vi "X_C_4352_15.vi"(0 "ek":dbl format="%#_13g", 2 "length":i32=15, 3 "q":dbl[](array[numeric])=[1.0, 1.0, 1.0, 1.0, 1.0, 1.0, 1.0, 1.0, 1.0, 1.0, 1.0, 1.0, 1.0, 1.0, 1.0] format="%#_13g") -> (5 "uk":dbl format="%#_13g")   [LabVIEW 2015]
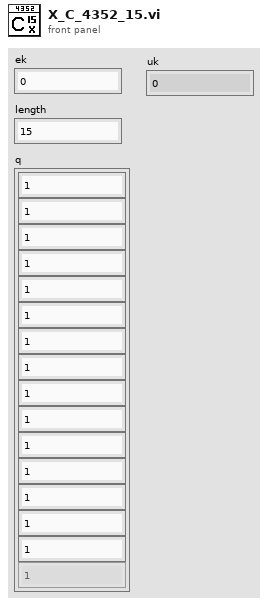
[diagram p1: front panel]
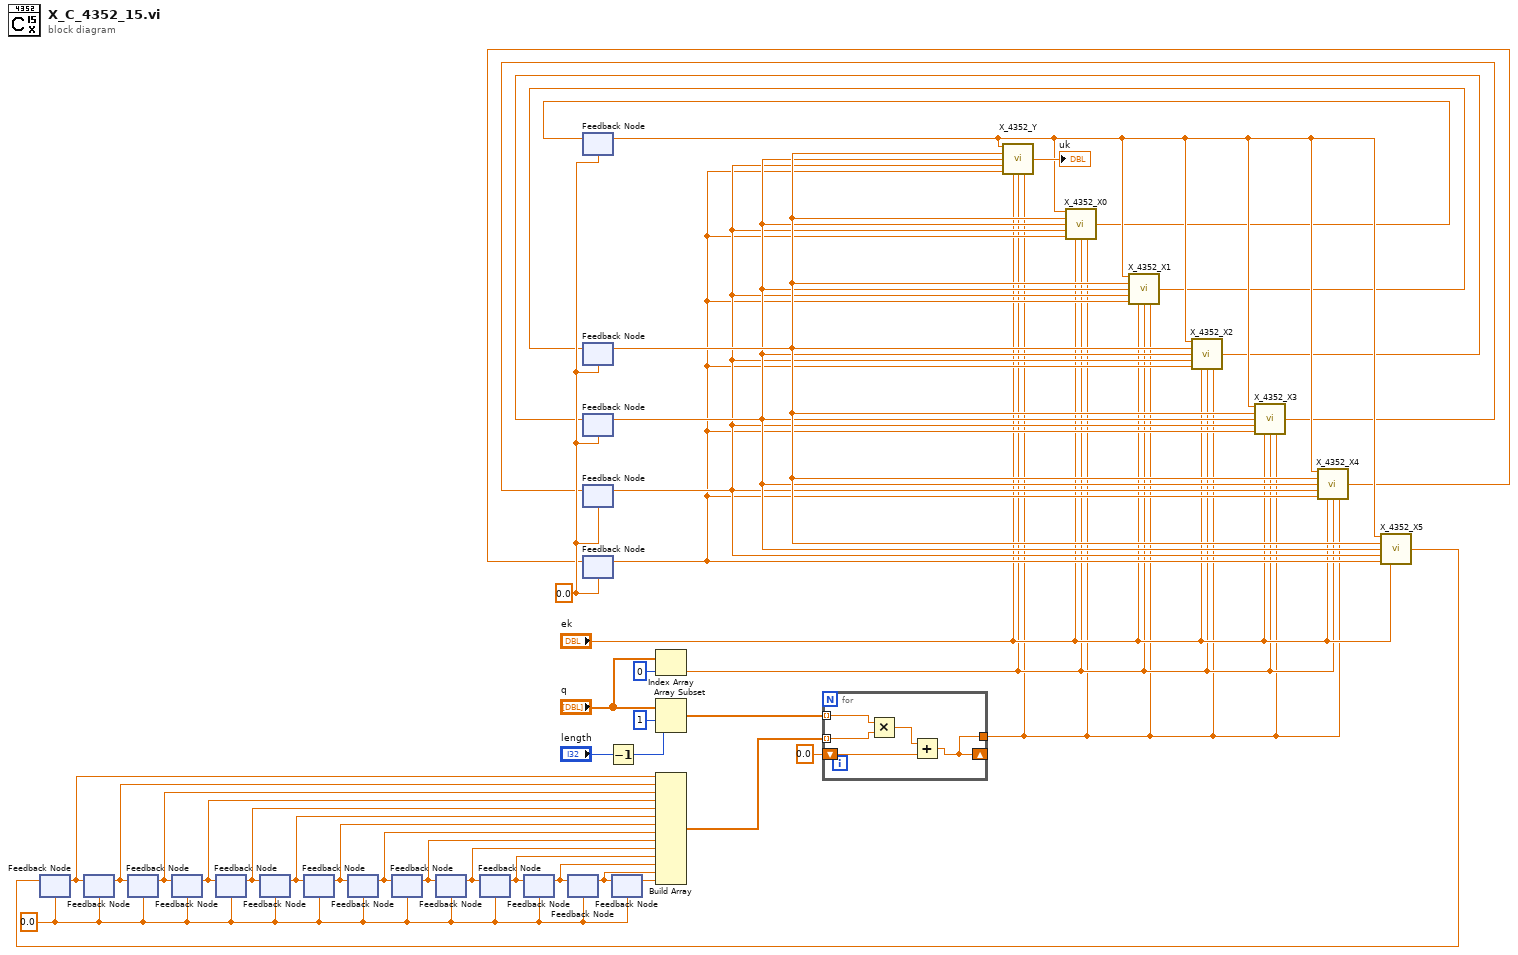
[diagram p0: block diagram]
diagram:
  w17 = 0.0
  w32 = 0.0
  n1 = feedback #1(w17) -> (w18:dbl)
  n2 = feedback #2(w17) -> (w19:dbl)
  n3 = feedback-in #2(w18) -> ()
  n4 = feedback #3(w17) -> (w20:dbl)
  n5 = feedback-in #3(w19) -> ()
  n6 = feedback #4(w17) -> (w21:dbl)
  n7 = feedback-in #4(w20) -> ()
  n8 = feedback #5(w17) -> (w22:dbl)
  n9 = feedback-in #5(w21) -> ()
  n10 = feedback #6(w17) -> (w23:dbl)
  n11 = feedback-in #6(w22) -> ()
  n12 = feedback #7(w17) -> (w24:dbl)
  n13 = feedback-in #7(w23) -> ()
  n14 = feedback #8(w17) -> (w25:dbl)
  n15 = feedback-in #8(w24) -> ()
  n16 = feedback #9(w17) -> (w26:dbl)
  n17 = feedback-in #9(w25) -> ()
  n18 = feedback #10(w17) -> (w27:dbl)
  n19 = feedback-in #10(w26) -> ()
  n20 = feedback #11(w17) -> (w28:dbl)
  n21 = feedback-in #11(w27) -> ()
  n22 = feedback #12(w17) -> (w29:dbl)
  n23 = feedback-in #12(w28) -> ()
  n24 = feedback #13(w17) -> (w30:dbl)
  n25 = feedback-in #13(w29) -> ()
  n26 = feedback #14(w32) -> (w14:dbl)
  n27 = feedback #15(w32) -> (w13:dbl)
  n28 = feedback #16(w32) -> (w12:dbl)
  n29 = feedback #17(w32) -> (w11:dbl)
  n30 = feedback #18(w32) -> (w10:dbl)
  n31 = Decrement(x="length") -> (x-1=w33:i32)
  n32 = feedback #19(w17) -> (w31:dbl)
  n33 = feedback-in #19(w30) -> ()
  n34 = Index Array(array="q", index=0) -> (element=w3:dbl)
  n35 = Array Subset(array="q", index=1, length=w33) -> (w34:dbl[])
  n36 = Build Array(w18, w19, w20, w21, w22, w23, w24, w25, w26, w27, w28, w29, w30, w31) -> (w16:dbl[])
  n37 = for {
    tunnel: w16 -> [w43] mode=indexing
    tunnel: w34 -> [w44] mode=indexing
    shift-right: [w40] -> _
    shift-left: 0.0 -> [w41]
    tunnel: [w40] -> w2
    n38 = Multiply(x=w44, y=w43) -> (x*y=w42:dbl)
    n39 = Add(x=w42, y=w41) -> (x+y=w40:dbl)
  }
  n40 = call "X_4352_Y.vi"("x0"=w14, "x1"=w13, "x2"=w12, "x3"=w11, "x4"=w10, "e"="ek", "q0"=w3, "qzsum"=w2) -> ("Yout"=→"uk":dbl)  [unwired: 7 in]
  n41 = call "X_4352_X0.vi"("x0"=w14, "x1"=w13, "x2"=w12, "x3"=w11, "x4"=w10, "e"="ek", "q0"=w3, "qzsum"=w2) -> ("X0out"=w9:dbl)  [unwired: 7 in]
  n42 = feedback-in #14(w9) -> ()
  n43 = call "X_4352_X1.vi"("x0"=w14, "x1"=w13, "x2"=w12, "x3"=w11, "x4"=w10, "e"="ek", "q0"=w3, "qzsum"=w2) -> ("X1out"=w8:dbl)  [unwired: 7 in]
  n44 = feedback-in #15(w8) -> ()
  n45 = call "X_4352_X2.vi"("x0"=w14, "x1"=w13, "x2"=w12, "x3"=w11, "x4"=w10, "e"="ek", "q0"=w3, "qzsum"=w2) -> ("X2out"=w7:dbl)  [unwired: 7 in]
  n46 = feedback-in #16(w7) -> ()
  n47 = call "X_4352_X3.vi"("x0"=w14, "x1"=w13, "x2"=w12, "x3"=w11, "x4"=w10, "e"="ek", "q0"=w3, "qzsum"=w2) -> ("X3out"=w6:dbl)  [unwired: 7 in]
  n48 = feedback-in #17(w6) -> ()
  n49 = call "X_4352_X4.vi"("x0"=w14, "x1"=w13, "x2"=w12, "x3"=w11, "x4"=w10, "e"="ek", "q0"=w3, "qzsum"=w2) -> ("X4out"=w5:dbl)  [unwired: 7 in]
  n50 = feedback-in #18(w5) -> ()
  n51 = call "X_4352_X5.vi"("x0"=w14, "x1"=w13, "x2"=w12, "x3"=w11, "x4"=w10, "e"="ek") -> ("X5out"=w1:dbl)  [unwired: 9 in]
  n52 = feedback-in #1(w1) -> ()
